vi "SET_COMP_n.vi"(2 "execute":bool, 7 "COMP values":cdb[](array[numeric]), 11 "error in (no error)":errorcluster) -> (4 "function return":string, 15 "error out":errorcluster)   [LabVIEW 2017, in "ZBOX_IS.lvlib"]
uses:
  ZBOX_IS.lvlib
panel:
  out "BytePtr":u8[](array[numeric])
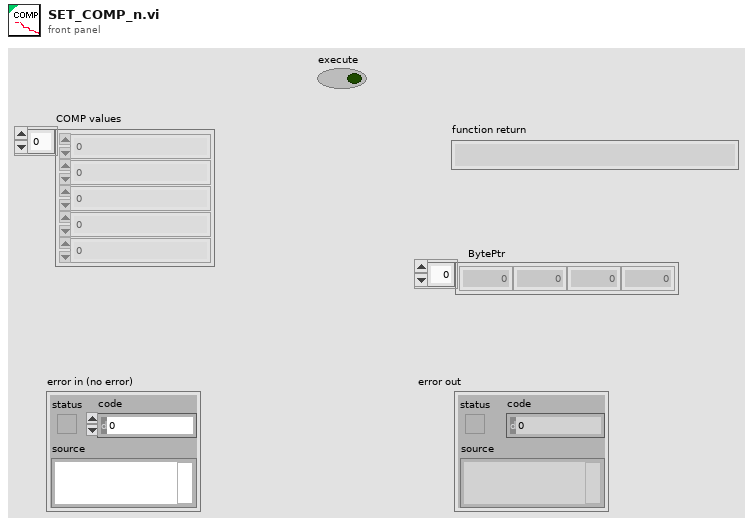
[diagram p1: front panel]
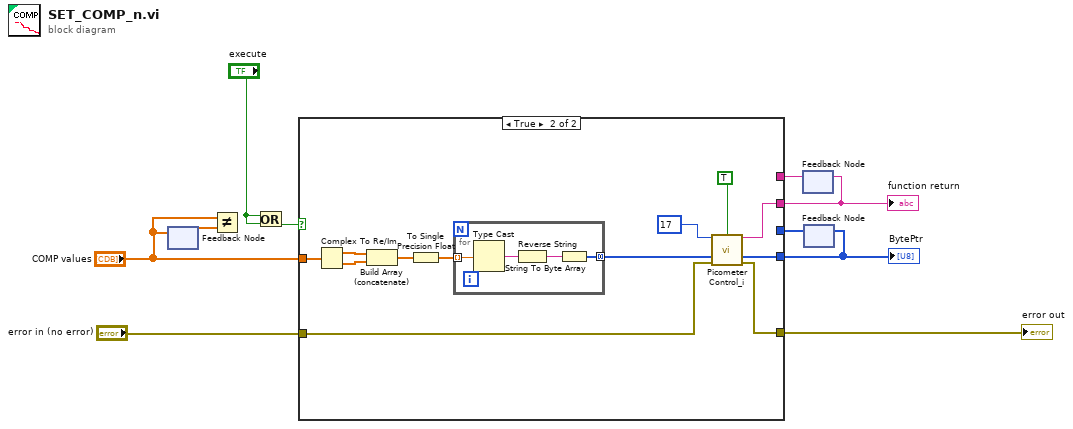
[diagram p0: block diagram]
diagram:
  n1 = feedback #1() -> (w8:cdb[])  [unwired: 1 in]
  n2 = feedback-in #1("COMP values") -> ()
  n3 = Not Equal?(x="COMP values", y=w8) -> ()  [unwired: 1 out]
  n4 = Or(x="execute", y="execute") -> (x .or. y?=w2:bool)
  n5 = feedback #2() -> (w4:string)  [unwired: 1 in]
  n6 = feedback #3() -> (w3:u8[])  [unwired: 1 in]
  n7 = case shown="True" w2 {
    tunnel: "error in (no error)" -> [w11 w25]
    tunnel: [w11 w24] -> w9
    tunnel: "COMP values" -> [_ w23]
    tunnel: [w13 w22] -> w6
    tunnel: [w12 w21] -> w5
    tunnel: w4 -> [w13 _]
    tunnel: w3 -> [w12 _]
    frame False {
    }
    frame True {
      n8 = Complex To Re/Im(x + iy=w23) -> (x=w19:dbl[], y=w18:dbl[])
      n9 = Build Array (concatenate)(w19, w18) -> (w17:dbl[])
      n10 = To Single Precision Float(number=w17) -> (single precision float=w16:sgl[])
      n11 = for {
        tunnel: w16 -> [w29] mode=indexing
        tunnel: [w27] -> w15 mode=concatenating
        n12 = Type Cast(x=w29) -> (*(type *) &x=w26:string)  [unwired: 1 in]
        n13 = Reverse String(1:w26) -> (0:w28:string)
        n14 = String To Byte Array(string=w28) -> (unsigned byte array=w27:u8[])
      }
      n15 = call "Picometer Control_i.vi"("Cmd"=u8 17, "execute"=TRUE, "BytePtr"=w15, "error in (no error)"=w25) -> ("function return"=w22:string, "BytePtr"=w21:u8[], "error out"=w24:errorcluster)  [unwired: 7 in, 2 out]
    }
  }
  "error out" <- w9
  "function return" <- w6
  "BytePtr" <- w5
  n16 = feedback-in #2(w6) -> ()
  n17 = feedback-in #3(w5) -> ()
